vi "Write IRead Voltage from Channel.vi"(8 "error in (no error)":errorcluster, 10 "IRead Voltage from Channel":refnum<class "IRead Voltage from Channel.lvclass">, 11 "Virtual Voltmeter in":refnum<class "Virtual Voltmeter.lvclass">) -> (0 "error out":errorcluster, 3 "Virtual Voltmeter out":refnum<class "Virtual Voltmeter.lvclass">)   [LabVIEW 2023, in "Voltmeter.lvlib" / "Virtual Voltmeter.lvlib" / "Virtual Voltmeter.lvclass"]
uses:
  Virtual Voltmeter.lvclass
  Interfaces/IRead Voltage Multichannel/IRead Voltage from Channel.lvclass
  Virtual Voltmeter.lvclass/Virtual Voltmeter.ctl
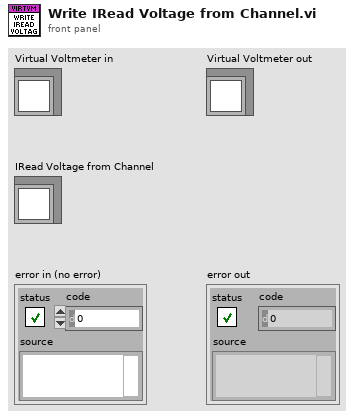
[diagram p1: front panel]
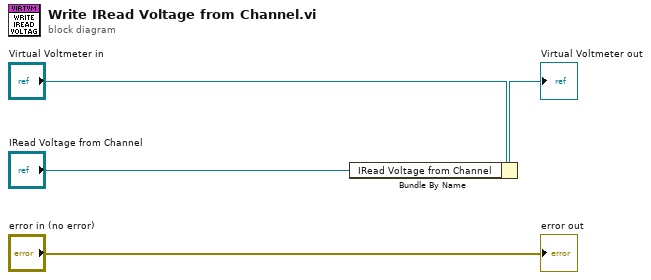
[diagram p0: block diagram]
diagram:
  n1 = Bundle By Name(cluster="Virtual Voltmeter in", "IRead Voltage from Channel"="IRead Voltage from Channel") -> (→"Virtual Voltmeter out":refnum<class "Virtual Voltmeter.lvclass">)
  "error out" <- "error in (no error)"
